vi "Scripting_Apply New VI Tools-Options Settings.vi"(8 "error in (no error)":errorcluster, 11 "VI Refnum":refnum<vi>) -> (0 "error out":errorcluster, 3 "dup VI Refnum":refnum<vi>)   [LabVIEW 2020]
doc: "Applies the following Tools > Options settings to the VI specified by VI Refnum:\n\nDefault justification: subdiagram labels\nPlace structures with Auto Grow enabled\nPlace front panel terminals as icons\nEnable automatic error handling in new VIs\nSeparate compiled code from new files"
uses:
  <vilib>/Utility/traverseref.llb/TRef TravTarget.ctl
  <resource>/dialog/lvconfig.llb/LV Config Read Numeric (I32).vi
  <resource>/dialog/lvconfig.llb/LV Config Read Boolean.vi
  <vilib>/Utility/traverseref.llb/VI Scripting - Traverse.lvlib
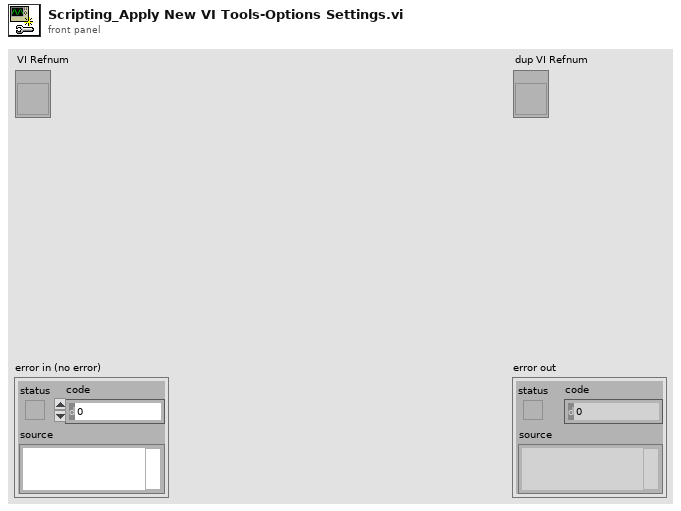
[diagram p1: front panel]
types:
  T1 = typedef "TRef TravTarget.ctl" = enum16{"FP", "BD", "Other"}
  T2 = enum32{"invalid VI type", "Standard VI", "Control VI", "Global VI", "Polymorphic VI", "Configuration VI", "SubSystem", "Facade VI", "Method VI", "Statechart Diagram VI"}
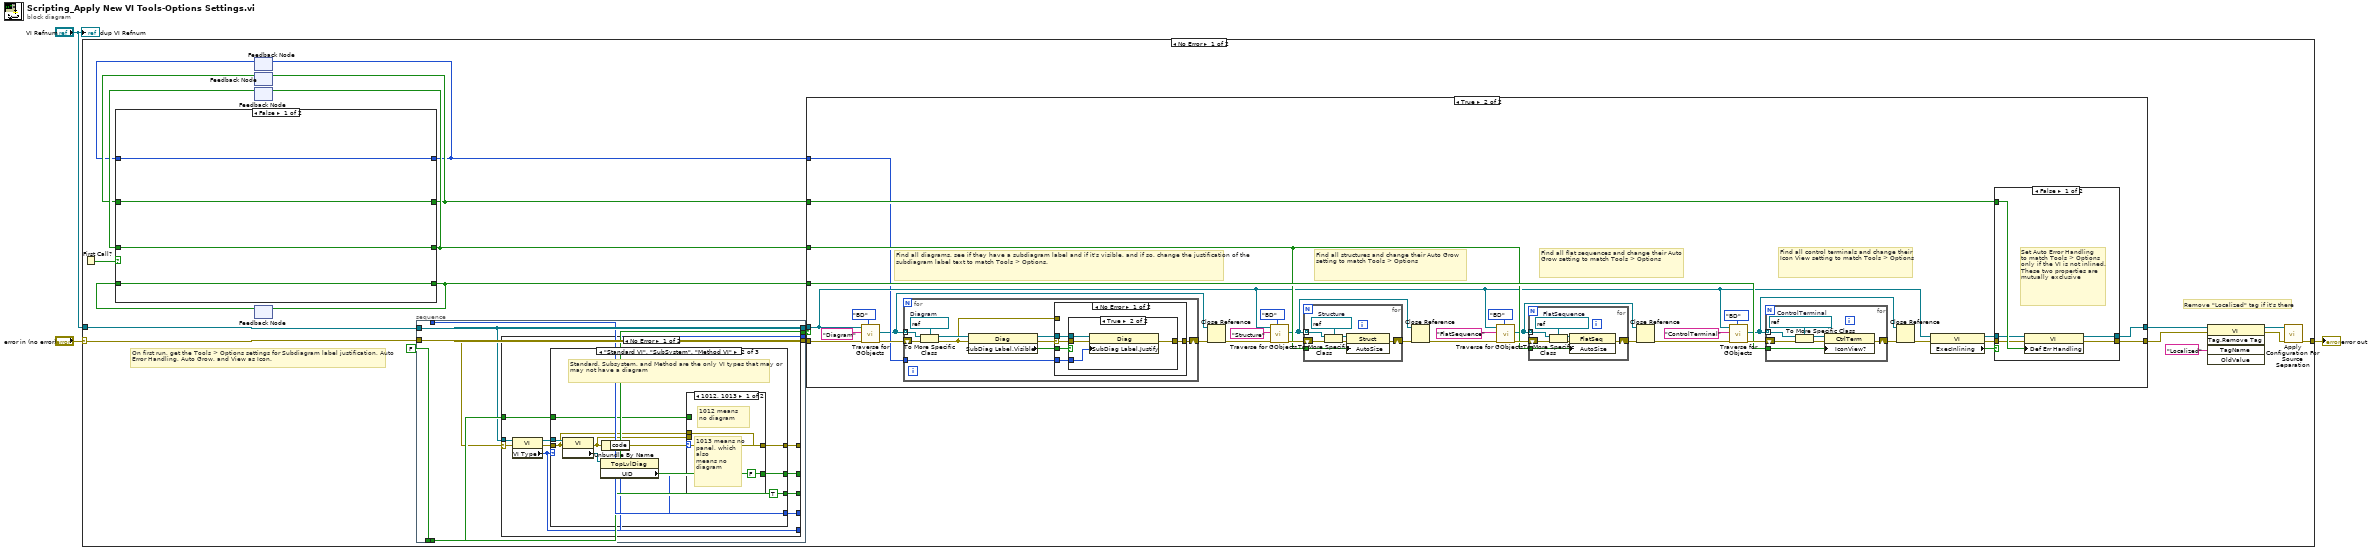
[diagram p0: block diagram]
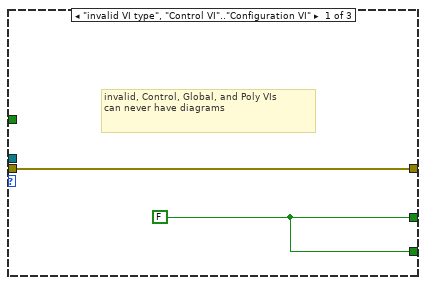
[diagram p2: hidden frame]
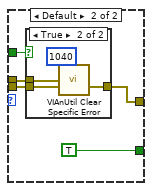
[diagram p3: hidden frame]
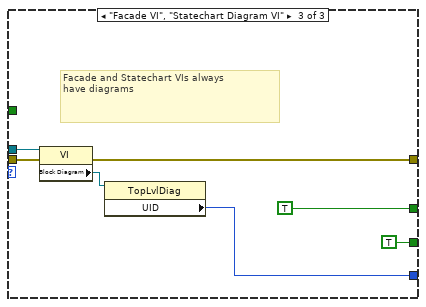
[diagram p5: hidden frame]
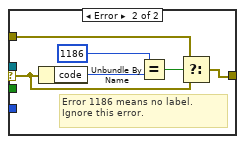
[diagram p9: hidden frame]
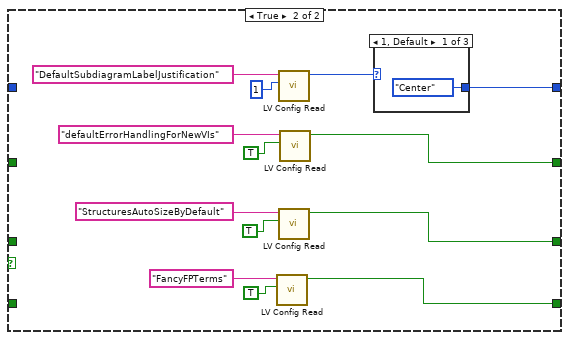
[diagram p11: hidden frame]
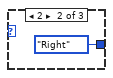
[diagram p12: hidden frame]
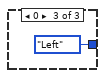
[diagram p13: hidden frame]
diagram:
  n1 = case shown="No Error" "error in (no error)" {
    selector: "error in (no error)" -> [w21 w186]
    tunnel: [w14 w186] -> w2
    tunnel: "VI Refnum" -> [w19 _]
    frame No Error {
      # "Remove \"Localized\" tag if it's there"
      # "On first run, get the Tools > Options settings for Subdiagram label justification, Auto Error Handling, Auto Grow, and View as Icon."
      n2 = First Call?() -> (First Call?: T/F=w24:bool)
      n3 = feedback #1() -> (w5:enum16{"Left", "Center", "Right"})  [unwired: 1 in]
      n4 = feedback #2() -> (w8:bool)  [unwired: 1 in]
      n5 = feedback #3() -> (w23:bool)  [unwired: 1 in]
      n6 = feedback #4() -> (w22:bool)  [unwired: 1 in]
      n7 = case shown="False" w24 {
        tunnel: [w169 w172] -> w17
        tunnel: [w168 w171] -> w16
        tunnel: w23 -> [w169 _]
        tunnel: w22 -> [w168 _]
        tunnel: [w167 w173] -> w7
        tunnel: w8 -> [w167 _]
        tunnel: [w166 w182] -> w6
        tunnel: w5 -> [w166 _]
        frame False {
        }
        frame True {
          n8 = call-poly <resource>:"LV Config Read.vi"("default value"=TRUE, "key"="FancyFPTerms") -> ("value"=w171:bool)  [unwired: 3 in, 2 out]
          n9 = call-poly <resource>:"LV Config Read.vi"("default value"=1 ("Subdiagram Label.Justification"), "key"="DefaultSubdiagramLabelJustification") -> ("value"=w170:i32)  [unwired: 3 in, 2 out]
          n10 = call-poly <resource>:"LV Config Read.vi"("default value"=TRUE, "key"="StructuresAutoSizeByDefault") -> ("value"=w172:bool)  [unwired: 3 in, 2 out]
          n11 = call-poly <resource>:"LV Config Read.vi"("default value"=TRUE, "key"="defaultErrorHandlingForNewVIs") -> ("value"=w173:bool)  [unwired: 3 in, 2 out]
          n12 = case shown="1, Default" w170 {
            tunnel: [enum16{"Left", "Center", "Right"}."Center" ("Subdiagram Label.Justification") enum16{"Left", "Center", "Right"}."Right" ("Subdiagram Label.Justification") enum16{"Left", "Center", "Right"}."Left" ("Subdiagram Label.Justification")] -> w182
            frame 1, Default {
            }
            frame 2 {
            }
            frame 0 {
            }
          }
        }
      }
      n13 = feedback-in #1(w6) -> ()
      n14 = feedback-in #2(w7) -> ()
      n15 = feedback-in #3(w17) -> ()
      n16 = feedback-in #4(w16) -> ()
      n17 = stacked-sequence {
        tunnel: [w26] -> w20
        tunnel: [w28] -> _
        tunnel: [w29] -> w15
        tunnel: [w27] -> w18
        tunnel: [w31] -> _
        tunnel: [w32] -> _
        tunnel: FALSE ("Clear 1040?") -> [w30]
        tunnel: w21 -> [w25]
        tunnel: w19 -> [w27]
        frame #0 {
          n18 = case shown="No Error" w25 {
            selector: w25 -> [w42 w74]
            tunnel: [w39 w74] -> w26
            tunnel: w27 -> [w41 _]
            tunnel: [w38 _] -> w28
            tunnel: [w36 _] -> w29
            tunnel: w30 -> [w35 _]
            tunnel: [w34 _] -> w31
            tunnel: [w33 _] -> w32
            frame No Error {
              n19 = property class="VI"(reference=w41, error in=w42) -> (reference out=w37:refnum<vi>, error out=w40:errorcluster, "VI Type"=w38:T2)
              n20 = case shown="\"Standard VI\", \"SubSystem\", \"Method VI\"" w38 {
                tunnel: w40 -> [w44 w51 w69]
                tunnel: [w44 w52 w70] -> w39
                tunnel: w37 -> [_ w54 w68]
                tunnel: [w43 w49 TRUE] -> w36
                tunnel: w35 -> [_ w47 _]
                tunnel: [w43 TRUE TRUE] -> w34
                tunnel: [_ w45 w67] -> w33
                frame "invalid VI type", "Control VI".."Configuration VI" {
                  w43 = FALSE
                  # "invalid, Control, Global, and Poly VIs\ncan never have diagrams"
                }
                frame "Standard VI", "SubSystem", "Method VI" {
                  # "Standard, Subsystem, and Method are the only VI types that may or may not have a diagram"
                  n21 = property class="VI"(reference=w54, error in=w51) -> (error out=w48:errorcluster, "Block Diagram"=w53:refnum<vi>)  [unwired: 1 out]
                  n22 = property class="TopLvlDiag"(reference=w53) -> ("UID"=w45:i32)  [unwired: 1 in, 2 out]
                  n23 = Unbundle By Name(w48) -> ("code"=w50:i32)
                  n24 = case shown="1012, 1013" w50 {
                    tunnel: [w56 w61] -> w52
                    tunnel: w51 -> [w56 w60]
                    tunnel: [FALSE TRUE] -> w49
                    tunnel: w48 -> [_ w58]
                    tunnel: w47 -> [_ w57]
                    frame 1012, 1013 {
                      # "1013 means no panel, which also\nmeans no diagram"
                      # "1012 means\nno diagram"
                    }
                    frame Default {
                      n25 = case shown="True" w57 {
                        tunnel: [w62 w66] -> w61
                        tunnel: w60 -> [_ w65]
                        tunnel: w58 -> [w62 w63]
                        frame False {
                        }
                        frame True {
                          n26 = call <vilib>:"VIAnUtil Clear Specific Error.vi"("Error of Interest"=1040, "error in (previous)"=w65, "error in (current)"=w63) -> ("error out"=w66:errorcluster)  [unwired: 12 out]
                        }
                      }
                    }
                  }
                }
                frame "Facade VI", "Statechart Diagram VI" {
                  # "Facade and Statechart VIs always\nhave diagrams"
                  n27 = property class="VI"(reference=w68, error in=w69) -> (error out=w70:errorcluster, "Block Diagram"=w71:refnum<vi>)  [unwired: 1 out]
                  n28 = property class="TopLvlDiag"(reference=w71) -> ("UID"=w67:i32)  [unwired: 1 in, 2 out]
                }
              }
            }
            frame Error {
            }
          }
        }
      }
      n29 = case shown="True" w15 {
        tunnel: w20 -> [w76 w93]
        tunnel: w18 -> [w75 w91]
        tunnel: [w76 w100] -> w13
        tunnel: w17 -> [_ w101]
        tunnel: w16 -> [_ w105]
        tunnel: [w75 w99] -> w11
        tunnel: w7 -> [_ w98]
        tunnel: w6 -> [_ w89]
        frame False {
          # "If the VI doesn't have a diagram, do nothing"
        }
        frame True {
          # "Find all diagrams, see if they have a subdiagram label and if it's visible, and if so, change the justification of the subdiagram label text to match Tools > Options."
          # "Find all flat sequences and change their Auto Grow setting to match Tools > Options"
          # "Find all control terminals and change their Icon View setting to match Tools > Options"
          # "Find all structures and change their Auto Grow setting to match Tools > Options"
          n30 = call <vilib>:"Traverse for GObjects.vi"("Traverse Target"=TRef_TravTarget."BD", "error in (no error)"=w93, "Class Name"="Diagram", "VI Refnum"=w91) -> ("error out"=w90:errorcluster, "References"=w86:refnum<vi>[])  [unwired: 4 in, 2 out]
          n31 = for {
            shift-right: [w112] -> w88
            shift-left: w90 -> [w121]
            tunnel: w86 -> [w120] mode=indexing
            tunnel: w89 -> [w113]
            w119 = refnum<vi> refnum  # Diagram
            n32 = To More Specific Class(target class=w119, reference=w120, error in=w121) -> (specific class reference=w118:refnum<vi>, error out=w114:errorcluster)
            n33 = property class="Diag"(reference=w118, error in=w114) -> (reference out=w115:refnum<vi>, error out=w117:errorcluster, "SubDiag Label.Visible"=w116:bool)
            n34 = case shown="No Error" w117 {
              selector: w117 -> [w125 w134]
              tunnel: w115 -> [w123 _]
              tunnel: w116 -> [w126 _]
              tunnel: w114 -> [_ w133]
              tunnel: [w124 w132] -> w112
              tunnel: w113 -> [w122 _]
              frame No Error {
                n35 = case shown="True" w126 {
                  tunnel: w125 -> [w127 w130]
                  tunnel: [w127 w131] -> w124
                  tunnel: w123 -> [_ w129]
                  tunnel: w122 -> [_ w128]
                  frame False {
                  }
                  frame True {
                    n36 = property class="Diag"(reference=w129, error in=w130, "SubDiag Label.Justify"=w128) -> (error out=w131:errorcluster)  [unwired: 1 out]
                  }
                }
              }
              frame Error {
                # "Error 1186 means no label. Ignore this error."
                n37 = Unbundle By Name(w134) -> ("code"=w137:i32)
                n38 = Equal?(x=1186, y=w137) -> (x = y?=w135:bool)
                n39 = Select(t=w133, s=w135, f=w134) -> (s? t:f=w132:errorcluster)
              }
            }
          }
          n40 = Close Reference(reference=w86, error in (no error)=w88) -> (error out=w87:errorcluster)
          n41 = call <vilib>:"Traverse for GObjects.vi"("Traverse Target"=TRef_TravTarget."BD", "error in (no error)"=w87, "Class Name"="Structure", "VI Refnum"=w91) -> ("error out"=w109:errorcluster, "References"=w83:refnum<vi>[])  [unwired: 4 in, 2 out]
          n42 = for {
            shift-right: [w159] -> w85
            shift-left: w109 -> [w165]
            tunnel: w83 -> [w164] mode=indexing
            tunnel: w101 -> [w160]
            w163 = refnum<vi> refnum  # Structure
            n43 = To More Specific Class(target class=w163, reference=w164, error in=w165) -> (specific class reference=w161:refnum<vi>, error out=w162:errorcluster)
            n44 = property class="Struct"(reference=w161, error in=w162, "AutoSize"=w160) -> (error out=w159:errorcluster)  [unwired: 1 out]
          }
          n45 = Close Reference(reference=w83, error in (no error)=w85) -> (error out=w84:errorcluster)
          n46 = call <vilib>:"Traverse for GObjects.vi"("Traverse Target"=TRef_TravTarget."BD", "error in (no error)"=w84, "Class Name"="FlatSequence", "VI Refnum"=w91) -> ("error out"=w104:errorcluster, "References"=w80:refnum<vi>[])  [unwired: 4 in, 2 out]
          n47 = for {
            shift-right: [w145] -> w82
            shift-left: w104 -> [w151]
            tunnel: w80 -> [w150] mode=indexing
            tunnel: w101 -> [w146]
            w149 = refnum<vi> refnum  # FlatSequence
            n48 = To More Specific Class(target class=w149, reference=w150, error in=w151) -> (specific class reference=w147:refnum<vi>, error out=w148:errorcluster)
            n49 = property class="FlatSeq"(reference=w147, error in=w148, "AutoSize"=w146) -> (error out=w145:errorcluster)  [unwired: 1 out]
          }
          n50 = Close Reference(reference=w80, error in (no error)=w82) -> (error out=w81:errorcluster)
          n51 = call <vilib>:"Traverse for GObjects.vi"("Traverse Target"=TRef_TravTarget."BD", "error in (no error)"=w81, "Class Name"="ControlTerminal", "VI Refnum"=w91) -> ("error out"=w106:errorcluster, "References"=w77:refnum<vi>[])  [unwired: 4 in, 2 out]
          n52 = for {
            tunnel: w105 -> [w153]
            tunnel: w77 -> [w157] mode=indexing
            shift-right: [w152] -> w79
            shift-left: w106 -> [w158]
            w156 = refnum<vi> refnum  # ControlTerminal
            n53 = To More Specific Class(target class=w156, reference=w157, error in=w158) -> (specific class reference=w154:refnum<vi>, error out=w155:errorcluster)
            n54 = property class="CtrlTerm"(reference=w154, error in=w155, "IconView?"=w153) -> (error out=w152:errorcluster)  [unwired: 1 out]
          }
          n55 = Close Reference(reference=w77, error in (no error)=w79) -> (error out=w78:errorcluster)
          n56 = property class="VI"(reference=w91, error in=w78) -> (reference out=w97:refnum<vi>, error out=w96:errorcluster, "ExecInlining"=w95:bool)
          n57 = case shown="False" w95 {
            tunnel: [w142 w143] -> w100
            tunnel: [w141 w144] -> w99
            tunnel: w98 -> [w140 _]
            tunnel: w97 -> [w139 w144]
            tunnel: w96 -> [w138 w143]
            frame False {
              # "Set Auto Error Handling\nto match Tools > Options only if the VI is not inlined. These two properties are mutually exclusive"
              n58 = property class="VI"(reference=w139, error in=w138, "Def Err Handling"=w140) -> (reference out=w141:refnum<vi>, error out=w142:errorcluster)
            }
            frame True {
            }
          }
        }
      }
      n59 = invoke class="VI" method="Tag.Remove Tag"(reference=w11, error in=w13, "TagName"="Localized" ("Tag Name")) -> (reference out=w12:refnum<vi>, error out=w10:errorcluster)  [unwired: 2 in, 3 out]
      n60 = call <vilib>:"Apply Configuration For Source Separation.vi"("error in (no error)"=w10, "VI in"=w12) -> ("error out"=w14:errorcluster)  [unwired: 8 in, 1 out]
    }
    frame Error {
    }
  }
  "error out" <- w2
  "dup VI Refnum" <- "VI Refnum"
